vi "Destroy OOB Communications.vi"(8 "error in (no error)":errorcluster, 11 "CIFTemplatePlugin in":refnum<class "Template_Plugin.lvclass">) -> (0 "error out":errorcluster, 3 "CIFTemplatePlugin out":refnum<class "Template_Plugin.lvclass">)   [LabVIEW 2021, in "Template_Plugin.lvclass"]
uses:
  Template_Plugin.lvclass
  Template_Plugin.lvclass/Template_Plugin.ctl
  <vilib>/CIF Foundation/CIF CIPC/CIF_NI_CIPC.lvlib
  Common/Typedef/OOB Comm/To Main DVR Data.ctl
  Common/Template_Common.lvlib
  Common/Typedef/OOB Comm/To gRPC DVR Data.ctl
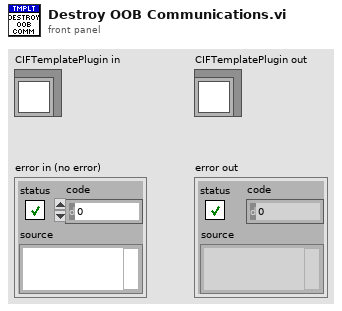
[diagram p1: front panel]
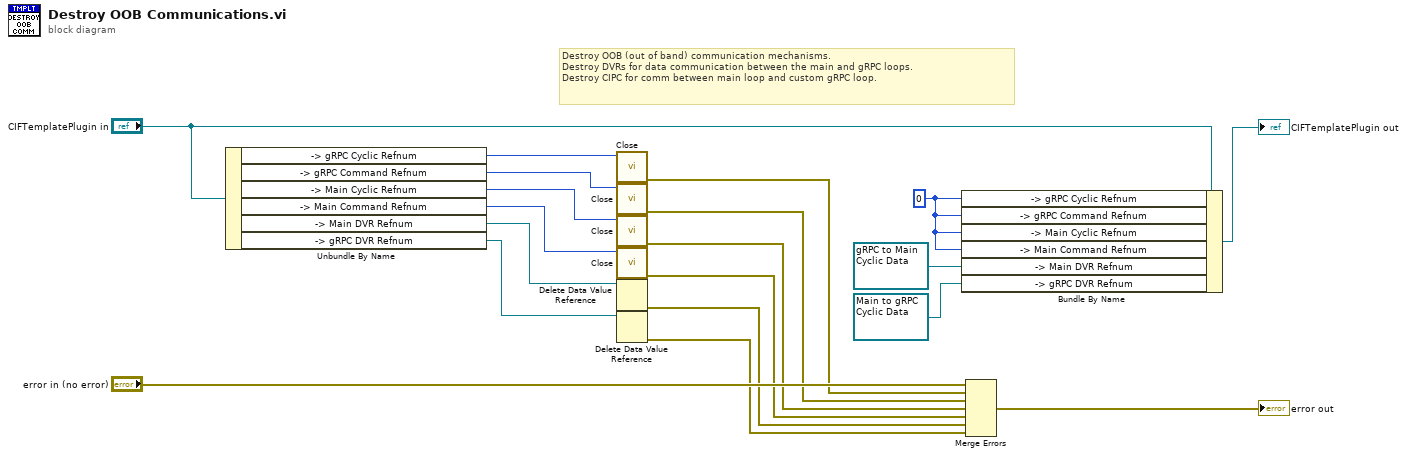
[diagram p0: block diagram]
diagram:
  w3 = u64 0 ("-> gRPC Comm.-> gRPC Cyclic Refnum")
  # "Destroy OOB (out of band) communication mechanisms.\nDestroy DVRs for data communication between the main and gRPC loops. \nDestroy CIPC for comm between main loop and custom gRPC loop."
  n1 = Unbundle By Name("CIFTemplatePlugin in") -> ("-> gRPC Cyclic Refnum"=w9:u64, "-> gRPC Command Refnum"=w10:u64, "-> Main Cyclic Refnum"=w11:u64, "-> Main Command Refnum"=w12:u64, "-> Main DVR Refnum"=w15:refnum<data-value>, "-> gRPC DVR Refnum"=w16:refnum<data-value>)
  n2 = call <vilib>:"Close.vi"("CIPC Reference"=w9) -> ("error out"=w7:errorcluster)  [unwired: 10 in]
  n3 = call <vilib>:"Close.vi"("CIPC Reference"=w10) -> ("error out"=w5:errorcluster)  [unwired: 10 in]
  n4 = call <vilib>:"Close.vi"("CIPC Reference"=w11) -> ("error out"=w6:errorcluster)  [unwired: 10 in]
  n5 = call <vilib>:"Close.vi"("CIPC Reference"=w12) -> ("error out"=w8:errorcluster)  [unwired: 10 in]
  n6 = Delete Data Value Reference(data value reference=w15) -> (error out=w13:errorcluster)  [unwired: 1 in, 1 out]
  n7 = Delete Data Value Reference(data value reference=w16) -> (error out=w14:errorcluster)  [unwired: 1 in, 1 out]
  n8 = Bundle By Name(cluster="CIFTemplatePlugin in", "-> gRPC Cyclic Refnum"=w3, "-> gRPC Command Refnum"=w3, "-> Main Cyclic Refnum"=w3, "-> Main Command Refnum"=w3, "-> Main DVR Refnum"=refnum<data-value> refnum ("-> Main Comm.-> Main DVR Refnum"), "-> gRPC DVR Refnum"=refnum<data-value> refnum ("-> gRPC Comm.-> gRPC DVR Refnum")) -> (→"CIFTemplatePlugin out":refnum<class "Template_Plugin.lvclass">)
  n9 = Merge Errors("error in (no error)", w7, w5, w6, w8, w13, w14) -> (→"error out":errorcluster)
